vi "FX65.vi"(11 "Variables and Memory in":T1 {"GFX" format="%02x"}) -> (3 "Variables and Memory out":T1 {"GFX" format="%02x"})   [LabVIEW 2021]
uses:
  Controls/ClusterF.ctl
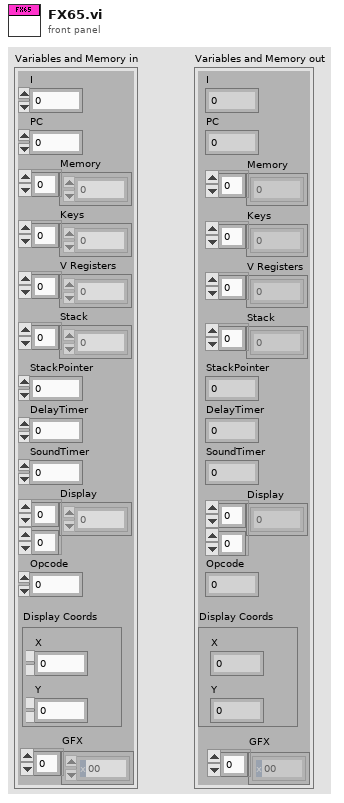
[diagram p1: front panel]
types:
  T1 = typedef "ClusterF.ctl" = cluster{"I":u16, "PC":u16, "Memory":u8[], "Keys":u8[], "V Registers":u8[], "Stack":u16[], "StackPointer":u16, "DelayTimer":u8, "SoundTimer":u8, "Display":u8[][], "Opcode":u16, "Display Coords":cluster{"X":u8, "Y":u8}, "GFX":u8[]}
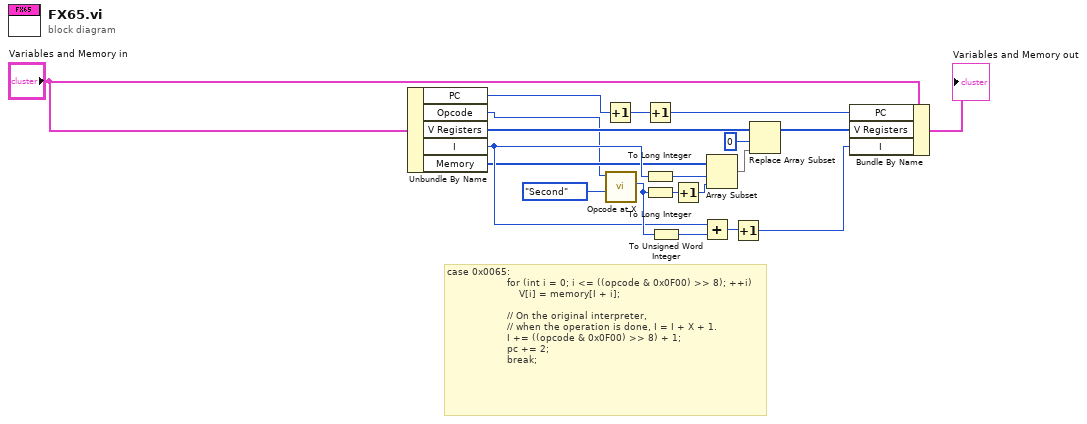
[diagram p0: block diagram]
diagram:
  # "case 0x0065:\n                    for (int i = 0; i <= ((opcode & 0x0F00) >> 8); ++i)\n                        V[i] = memory[I + i];\n\n                    // On the original interpreter,\n                    // when the operation is done, I = I + X + 1.\n                    I += ((opcode & 0x0F00) >> 8) + 1;\n                    pc += 2;\n                    break;"
  n1 = Unbundle By Name("Variables and Memory in") -> ("PC"=w11:u16, "Opcode"=w1:u16, "V Registers"=w4:u8[], "I"=w15:u16, "Memory"=w3:u8[])
  n2 = Increment(x=w11) -> (x+1=w10:u16)
  n3 = call "Opcode at X.vi"("X Position"=enum16{"First", "Second", "Third", "Fourth"}."Second", "Opcode"=w1) -> ("Opcode at X Position (U8)"=w16:u8)  [unwired: 9 in]
  n4 = Increment(x=w10) -> (x+1=w12:u16)
  n5 = To Long Integer(number=w15) -> (32bit integer=w13:i32)
  n6 = To Long Integer(number=w16) -> (32bit integer=w14:i32)
  n7 = To Unsigned Word Integer(number=w16) -> (unsigned 16bit integer=w17:u16)
  n8 = Increment(x=w14) -> (x+1=w20:i32)
  n9 = Add(x=w15, y=w17) -> (x+y=w18:u16)
  n10 = Array Subset(array=w3, index=w13, length=w20) -> (w6:u8[])
  n11 = Increment(x=w18) -> (x+1=w19:u16)
  n12 = Replace Array Subset(array=w4, new element=w6, index=0) -> (w9:u8[])
  n13 = Bundle By Name(cluster="Variables and Memory in", "PC"=w12, "V Registers"=w9, "I"=w19) -> (→"Variables and Memory out":T1)
